vi "Build Frame Script Core.vi"(8 "error in (no error)":errorcluster, 10 "Config Array":string[](array[string]), 11 "SPI Root Pattern Creator in":refnum<class "SPI Root Pattern Creator.lvclass">) -> (0 "error out":errorcluster, 2 "Pattern Script":string, 3 "SPI Root Pattern Creator out":refnum<class "SPI Root Pattern Creator.lvclass">)   [LabVIEW 2018, in "SPI Root Pattern Creator.lvlib" / "SPI Root Pattern Creator.lvclass"]
uses:
  SPI Root Pattern Creator.lvclass
  Interfaces/Protocol Interface.lvlibp/Interfaces/Protocol Interface/Protocol Interface.lvclass
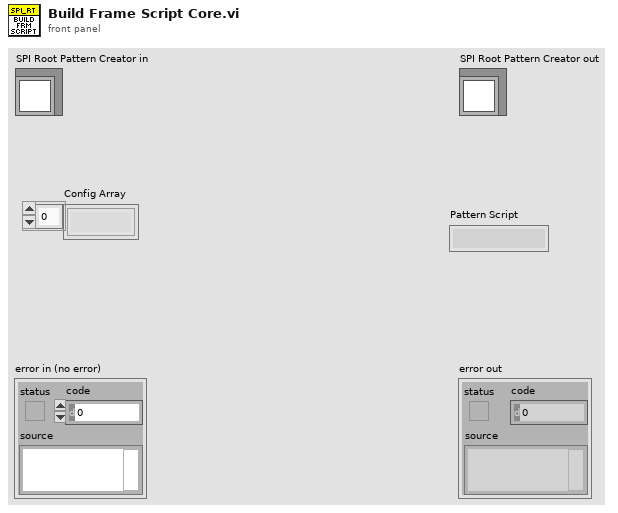
[diagram p1: front panel]
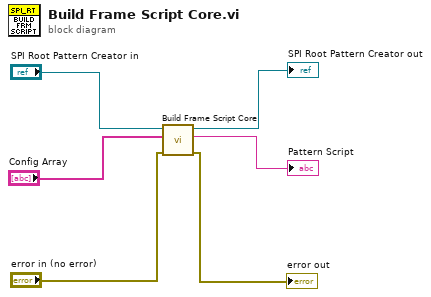
[diagram p0: block diagram]
diagram:
  n1 = call-parent "Build Frame Script Core.vi"("error in (no error)"="error in (no error)", "Config Array"="Config Array", "Protocol Interface in"="SPI Root Pattern Creator in") -> ("error out"=→"error out":errorcluster, "Pattern Script"=→"Pattern Script":string, "Protocol Interface out"=→"SPI Root Pattern Creator out":refnum<class "SPI Root Pattern Creator.lvclass">)  [unwired: 6 in]
